vi "myRIO_BRig_RT__Case_Exp_State_Enl1Pre__v3.vi"(7 "input_I_lick":bool, 8 "input_arrTrig":bool[](array[boolean]), 11 "input_dataCurrent":u16[](array[numeric])) -> (0 "output_l1_laserOn":bool, 1 "output_l1_laserEvent":bool, 3 "output_dataCurrent":u16[](array[numeric]), 4 "output_l2_laserEvent":bool, 5 "output_state":T1, 6 "output_l2_laserOn":bool)   [LabVIEW 2014]
uses:
  myRIO_BRig_RT__Case_Exp_stateList.ctl
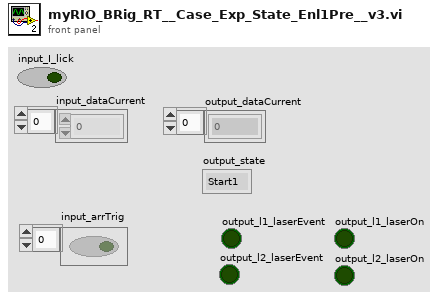
[diagram p1: front panel]
types:
  T1 = typedef "myRIO_BRig_RT__Case_Exp_stateList.ctl" = enum16{"Start1", "Start2", "Start3", "saveSettings1", "saveSettings2", "saveSettings3", "saveSettings4", "saveSettings_LC_ENL_l1", "saveSettings_LC_ENL_l2", "saveSettings_LC_Cue_l1", "saveSettings_LC_Cue_l2", "saveSettings6_LC_l1_Other", "SaveSettings6_LC_l2_Other", "setSettings_Audio", "setSettings_Laser", "initBlock_pre", "initBlock", "initBlock2", "initBlock_post", "initTrial_pre", "initTrial", "initTrial2", "initTrial3", "initTrial4", "initTrial_LC_ENL1", "initTrial_LC_Cue1", "initTrial_LC_Cue1_2", "initTrial_LC_Sel", "initTrial_post", "ENL1_pre", "ENL1", "ENL1_post", "ENL1Penalty_pre", "ENL1Penalty", "ENL2_pre", "ENL2", "ENL2Penalty_pre", "ENL2Penalty", "Cue1_pre", "Cue1", "Cue1_post", "Cue1Penalty_pre", "Cue1Penalty", "Cue2_pre", "Cue2", "Cue2Penalty_pre", "Cue2Penalty", "Selection_pre", "Selection", "Select_post", "SelectReward_pre", "SelectReward", "SelectRewardPost_pre", "SelectRewardPost", "SelectWrong_pre", "SelectWrong", "SelectWrong_post", "SelectTimeout_pre", "SelectTimeout", "SelectTimeout_post", "endTrial_pre", "endTrial1", "endTrial2", "endTrial3", "endTrial_post", "endBlock_pre", "endBlock", "endBlock_post", "endExp", "commConnect", "commUpload_pre", "commUpload_dataBlock", "commUpload_dataCurrent", "commUpload_dataExp", "commUpload_dataLC", "commUpload_dataTrial", "commUpload_post", "saveData_pre", "saveData_dataBlock", "saveData_dataCurrent", "saveData_dataExp", "saveData_dataLC", "saveData_dataTrial", "saveData_post", "empty_endBlock1", "empty_endBlock2", "empty_endTrial1", "empty_endTrial2", "empty_endTrial3", "empty_endTrial4", "empty_endTrial5", "dummyState", "dummyState_endBlock"}
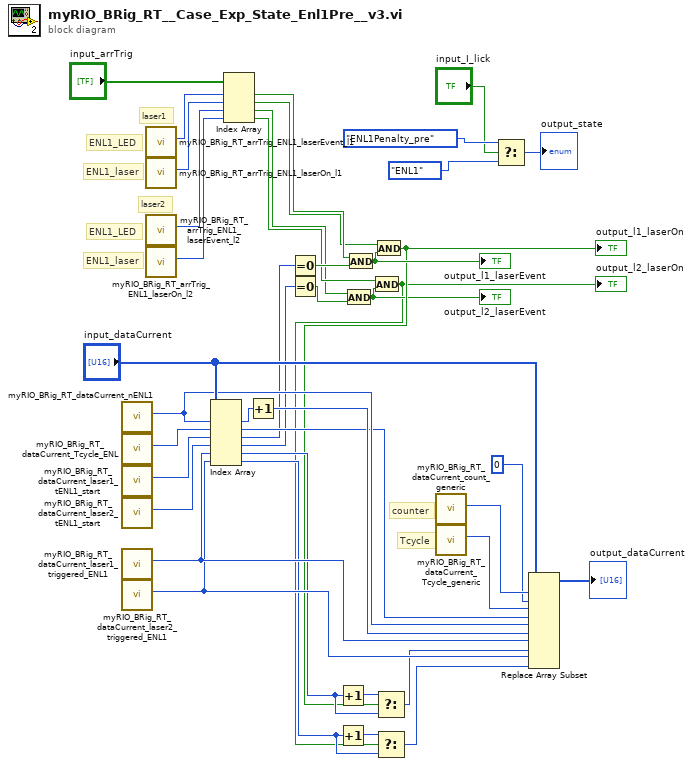
[diagram p0: block diagram]
diagram:
  # "ENL1_LED"
  # "ENL1_laser"
  # "ENL1_LED"
  # "ENL1_laser"
  # "laser2"
  # "laser1"
  # "Tcycle"
  # "counter"
  n1 = call "myRIO_BRig_RT_dataCurrent_nENL1.vi"() -> ("output_nENL1"=w33:i32)  [unwired: 11 in]
  n2 = call "myRIO_BRig_RT_dataCurrent_Tcycle_ENL.vi"() -> ("output_ENL"=w30:i32)  [unwired: 11 in]
  n3 = call "myRIO_BRig_RT_dataCurrent_laser1_tENL1_start.vi"() -> ("output_laser1_tENL1_start"=w29:i32)  [unwired: 11 in]
  n4 = call "myRIO_BRig_RT_dataCurrent_laser2_tENL1_start.vi"() -> ("output_laser2_tENL1_start"=w28:i32)  [unwired: 11 in]
  n5 = call "myRIO_BRig_RT_dataCurrent_laser1_triggered_ENL1.vi"() -> ("output_laser1_triggered_ENL1"=w19:i32)  [unwired: 11 in]
  n6 = call "myRIO_BRig_RT_dataCurrent_laser2_triggered_ENL1.vi"() -> ("output_laser2_triggered_ENL1"=w18:i32)  [unwired: 11 in]
  n7 = call "myRIO_BRig_RT_arrTrig_ENL1_laserEvent_l1.vi"() -> ("output_arrTrig_ENL1_laserEvent_l1"=w22:i32)  [unwired: 11 in]
  n8 = call "myRIO_BRig_RT_arrTrig_ENL1_laserOn_l1.vi"() -> ("output_arrTrig_ENL1_laserOn_l1"=w21:i32)  [unwired: 11 in]
  n9 = call "myRIO_BRig_RT_arrTrig_ENL1_laserEvent_l2.vi"() -> ("output_arrTrig_ENL1_laserEvent_l2"=w23:i32)  [unwired: 11 in]
  n10 = call "myRIO_BRig_RT_arrTrig_ENL1_laserOn_l2.vi"() -> ("output_arrTrig_ENL1_laserOn_l2"=w24:i32)  [unwired: 11 in]
  n11 = Index Array(array="input_dataCurrent", index #1=w33, index #2=w30, index #3=w29, index #4=w28, index #5=w19, index #6=w18) -> (element #1=w32:u16, element #2=w27:u16, element #3=w26:u16, element #4=w25:u16, element #5=w15:u16, element #6=w14:u16)
  n12 = Index Array(array="input_arrTrig", index #1=w22, index #2=w21, index #3=w23, index #4=w24) -> (element #1=w10:bool, element #2=w8:bool, element #3=w3:bool, element #4=w4:bool)
  n13 = Increment(x=w32) -> (x+1=w31:u16)
  n14 = Equal To 0?(x=w26) -> (x = 0?=w11:bool)
  n15 = Equal To 0?(x=w25) -> (x = 0?=w2:bool)
  n16 = Increment(x=w15) -> (x+1=w17:u16)
  n17 = Increment(x=w14) -> (x+1=w16:u16)
  n18 = And(x=w3, y=w2) -> (x .and. y?=w6:bool)
  "output_l2_laserEvent" <- w6
  n19 = And(x=w10, y=w11) -> (x .and. y?=w9:bool)
  "output_l1_laserEvent" <- w9
  n20 = And(x=w4, y=w6) -> (x .and. y?=w5:bool)
  "output_l2_laserOn" <- w5
  n21 = And(x=w8, y=w9) -> (x .and. y?=w7:bool)
  "output_l1_laserOn" <- w7
  n22 = Select(t=w17, s=w7, f=w15) -> (s? t:f=w13:u16)
  n23 = Select(t=w16, s=w5, f=w14) -> (s? t:f=w12:u16)
  n24 = call "myRIO_BRig_RT_dataCurrent_count_generic.vi"() -> ("output_count_generic"=w36:i32)  [unwired: 11 in]
  n25 = call "myRIO_BRig_RT_dataCurrent_Tcycle_generic.vi"() -> ("output_Tcycle_generic"=w35:i32)  [unwired: 11 in]
  n26 = Select(t=myRIO_BRig_RT__Case_Exp_stateList."ENL1Penalty_pre" ("Enum"), s="input_I_lick", f=myRIO_BRig_RT__Case_Exp_stateList."ENL1" ("Enum")) -> (s? t:f=→"output_state":T1)
  n27 = Replace Array Subset(array="input_dataCurrent", new element #1=u16 0 ("new element/subarray"), index #1=w36, new element #2=w27, index #2=w35, new element #3=w31, index #3=w33, new element #4=w13, index #4=w19, new element #5=w12, index #5=w18) -> (→"output_dataCurrent":u16[])
